vi "onGetLeafName.vi"(8 "error in (no error)":errorcluster, 11 "Leaf.Properties in":refnum<class "Leaf.Properties.lvclass">) -> (0 "error out":errorcluster, 2 "Name":string, 3 "Leaf.Properties out":refnum<class "Leaf.Properties.lvclass">)   [LabVIEW 2021, in "Banana.Caraya.lvlib" / "Leaf.Properties.lvclass"]
uses:
  Leaf.Properties.lvclass
  Leaf.Properties.lvclass/Leaf.Properties.ctl
  <vilib>/addons/_JKI Toolkits/Caraya/classes/Properties/Properties.lvclass
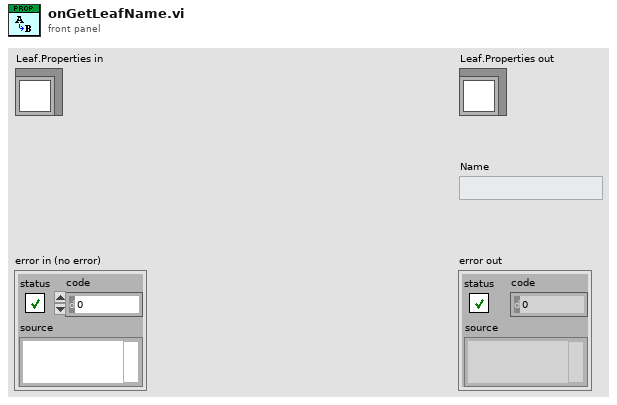
[diagram p1: front panel]
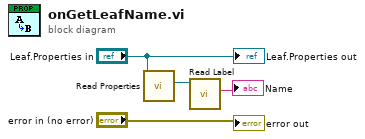
[diagram p0: block diagram]
diagram:
  n1 = call "Read Properties.vi"("Leaf.Properties in"="Leaf.Properties in") -> ("Properties"=w3:refnum<class "Properties.lvclass">)  [unwired: 9 in, 1 out]
  n2 = call <vilib>:"Read Label.vi"("Properties in"=w3) -> ("Test Label"=→"Name":string)  [unwired: 9 in, 1 out]
  "error out" <- "error in (no error)"
  "Leaf.Properties out" <- "Leaf.Properties in"
